vi "继保虚遥信转.vi"(1 "虚遥信":bool[](array[boolean])=[FALSE, FALSE, FALSE, FALSE, FALSE, FALSE, FALSE, FALSE, FALSE, FALSE, FALSE, FALSE, FALSE, FALSE, FALSE, FALSE] caption="虚遥信in") -> (0 "虚遥信out":T1)   [LabVIEW 2015]
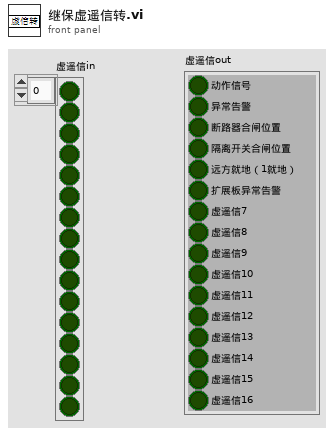
[diagram p1: front panel]
types:
  T1 = cluster{"动作信号":bool, "异常告警":bool, "断路器合闸位置":bool, "隔离开关合闸位置":bool, "远方就地（1就地）":bool, "扩展板异常告警":bool, "虚遥信7":bool, "虚遥信8":bool, "虚遥信9":bool, "虚遥信10":bool, "虚遥信11":bool, "虚遥信12":bool, "虚遥信13":bool, "虚遥信14":bool, "虚遥信15":bool, "虚遥信16":bool}
  T2 = cluster{"Boolean":bool, "Boolean":bool, "Boolean":bool, "Boolean":bool, "Boolean":bool, "Boolean":bool, "Boolean":bool, "Boolean":bool, "Boolean":bool, "Boolean":bool, "Boolean":bool, "Boolean":bool, "Boolean":bool, "Boolean":bool, "Boolean":bool, "Boolean":bool}
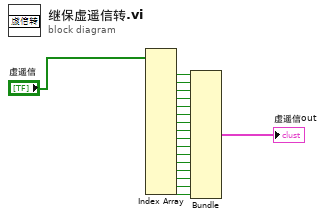
[diagram p0: block diagram]
diagram:
  n1 = Index Array(array="虚遥信") -> (element #1=w18:bool, element #2=w17:bool, element #3=w16:bool, element #4=w15:bool, element #5=w14:bool, element #6=w13:bool, element #7=w12:bool, element #8=w11:bool, element #9=w10:bool, element #10=w9:bool, element #11=w8:bool, element #12=w7:bool, element #13=w5:bool, element #14=w4:bool, element #15=w3:bool, element #16=w2:bool)  [unwired: 16 in]
  n2 = Bundle("Boolean"=w18, "Boolean"=w17, "Boolean"=w16, "Boolean"=w15, "Boolean"=w14, "Boolean"=w13, "Boolean"=w12, "Boolean"=w11, "Boolean"=w10, "Boolean"=w9, "Boolean"=w8, "Boolean"=w7, "Boolean"=w5, "Boolean"=w4, "Boolean"=w3, "Boolean"=w2) -> (→"虚遥信out":T2)  [unwired: 1 in]
